vi "Insert into Childs SubPanel.vi"(8 "error in (no error)":errorcluster, 10 "UI VI Ref":refnum<vi>, 11 "ViewableActorEncaps in":refnum<class "ViewableActorEncaps.lvclass">) -> (0 "error out":errorcluster, 3 "ViewableActorEncaps out":refnum<class "ViewableActorEncaps.lvclass">)   [LabVIEW 2020, in "ViewableActor.lvlib" / "ViewableActorEncaps.lvclass"]
uses:
  ViewableActorEncaps.lvclass
  ViewableActorEncaps.lvclass/ViewableActorEncaps.ctl
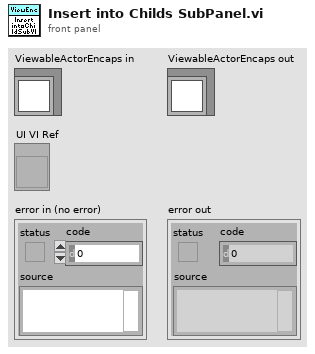
[diagram p1: front panel]
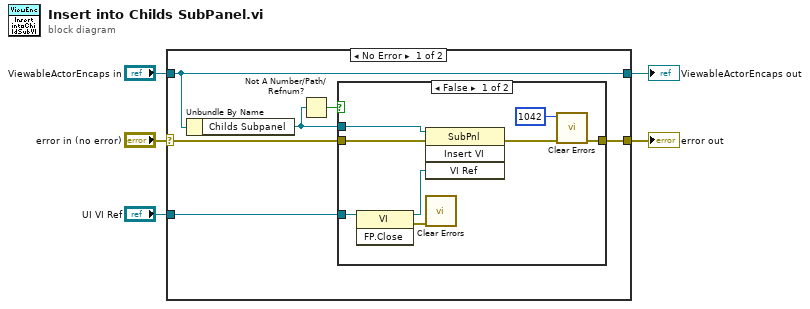
[diagram p0: block diagram]
diagram:
  n1 = case shown="No Error" "error in (no error)" {
    selector: "error in (no error)" -> [w10 w22]
    tunnel: [w8 w22] -> w4
    tunnel: [w11 w21] -> w2
    tunnel: "ViewableActorEncaps in" -> [w11 w21]
    tunnel: "UI VI Ref" -> [w9 _]
    frame No Error {
      n2 = Unbundle By Name(w11) -> ("Childs Subpanel"=w6:refnum<vi>)
      n3 = Not A Number/Path/Refnum?(number/path/refnum=w6) -> (NaN/Path/Refnum?=w7:bool)
      n4 = case shown="False" w7 {
        tunnel: w10 -> [w19 w20]
        tunnel: w9 -> [w16 _]
        tunnel: w6 -> [w14 _]
        tunnel: [w13 w20] -> w8
        frame False {
          n5 = invoke class="VI" method="FP.Close"(reference=w16) -> (reference out=w15:refnum<vi>, error out=w17:errorcluster)  [unwired: 2 in, 1 out]
          n6 = invoke on="Invoke Node" class="SubPnl" method="Insert VI"(reference=w14, error in=w19, "VI Ref"=w15) -> (error out=w18:errorcluster)  [unwired: 1 in, 3 out]
          n7 = call <vilib>:"Clear Errors.vi"("error in (no error)"=w17) -> ()  [unwired: 5 in, 2 out]
          n8 = call <vilib>:"Clear Errors.vi"("error in (no error)"=w18, "specific error code to clear (0: all)"=1042) -> ("error out"=w13:errorcluster)  [unwired: 4 in, 1 out]
        }
        frame True {
        }
      }
    }
    frame Error {
    }
  }
  "error out" <- w4
  "ViewableActorEncaps out" <- w2
